vi "Create Tags.vi"(8 "error in (no error)":errorcluster, 9 "Module Tags Array Cluster":T1, 10 "folder node ID":T14, 11 "Refnum in":T17) -> (0 "error out":errorcluster, 3 "Tags Array":T16(array[cluster]))   [LabVIEW 2018]
uses:
  <vilib>/OPCUA/controls/OPC UA Server Refnum.ctl
  <vilib>/OPCUA/controls/NodeId.ctl
  <vilib>/OPCUA/controls/OPC UA Variable Node Refnum.ctl
  Module Tags Array Cluster.ctl
  Feed Module/Controls/Feed Module Tag Names Cluster.ctl
  TT Module/Controls/TT Module Tag Names.ctl
  PT Module/Controls/PT Module Tag Names.ctl
  Pump Module Folder/Pump Module Tag Names Cluster.ctl
  Bronkhorst M14 Flow Meter/Tag Cluster.ctl
  TCU Module/TCU Module Folder/TCU Module Tag Names Cluster.ctl
  D-O Module Folder/D-O Module Tag Names Cluster.ctl
  Pressure Regulator Control Module/Pressure Regulator/Controls/4-20mA Module Tag Names Cluster.ctl
  OPC Module Tag Names.ctl
  Sonicator Module Folder/Feed Module/Controls/Sonicator Module Tag Names.ctl
  Agitator Class/Agitator Module Tag Names.ctl
  Centrifuge Module Folder/Centrifuge Module Tag Names Cluster.ctl
  <vilib>/OPCUA/controls/Data Type.ctl
  <vilib>/regexp/Match Regular Expression.xnode
  <vilib>/OPCUA/NI OPC UA Server.lvlib
  Feed Module/Feed Module.lvlib
  Pump Module Folder/Pump Module.lvlib
  Flow Module Folder/Flow Module.lvlib
  TCU Module/TCU Module Folder/TCU Module.lvlib
  Pressure Regulator Control Module/Pressure Regulator/4-20mA Module.lvlib
  Sonicator Module Folder/Sonicator Module.lvlib
  Agitator Module Folder/Agitator Module.lvlib
  PT Module/PT Module.lvlib
  TT Module/TT Module.lvlib
  D-O Module Folder/D-O Module.lvlib
  Centrifuge Module Folder/Centrifuge Module.lvlib
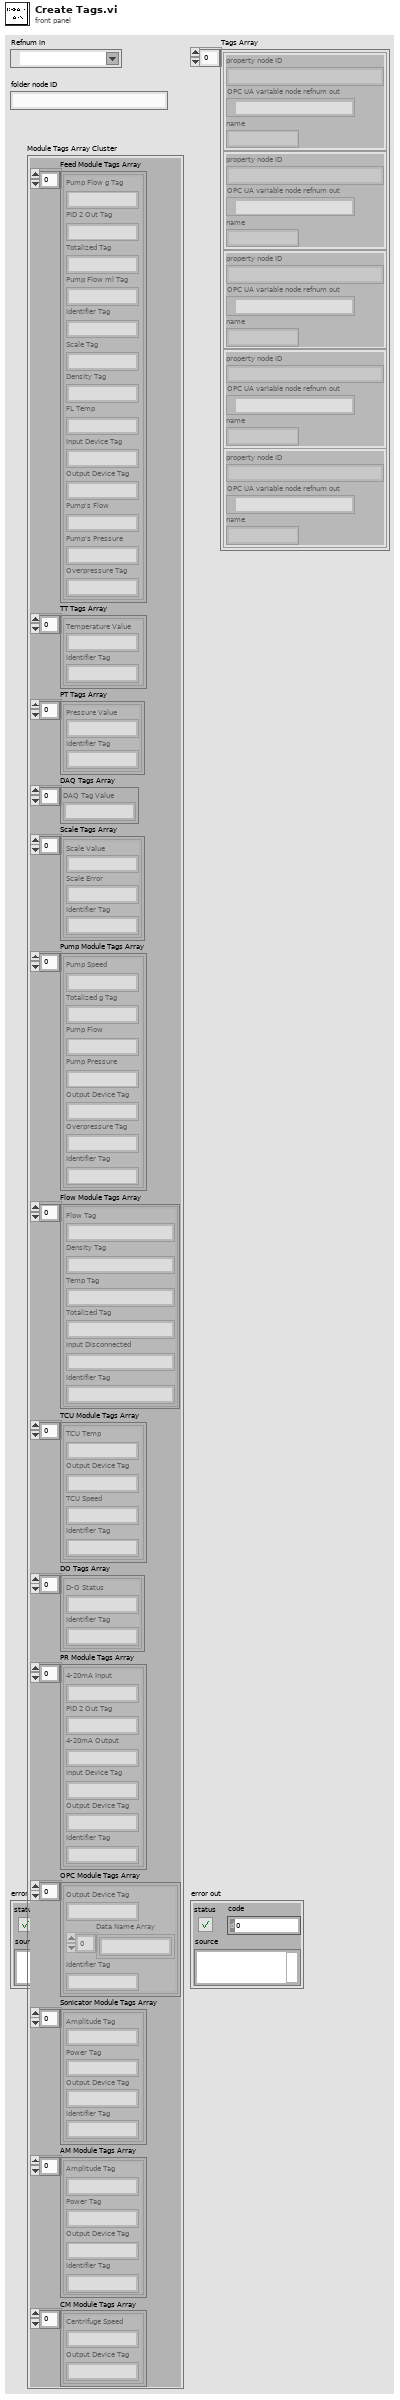
[diagram p1: front panel]
types:
  T1 = typedef "Module Tags Array Cluster.ctl" = cluster{"Feed Module Tags Array":T2[], "TT Tags Array":T3[], "PT Tags Array":T4[], "DAQ Tags Array":string[], "Scale Tags Array":cluster{"Scale Value":string, "Scale Error":string, "Identifier Tag":string}[], "Pump Module Tags Array":T5[], "Flow Module Tags Array":T6[], "TCU Module Tags Array":T7[], "DO Tags Array":T8[], "PR Module Tags Array":T9[], "OPC Module Tags Array":T10[], "Sonicator Module Tags Array":T11[], "AM Module Tags Array":T12[], "CM Module Tags Array":T13[]}
  T2 = typedef "Feed Module.lvlib/Feed Module Tag Names Cluster.ctl" = cluster{"Pump Flow g Tag":string, "PID 2 Out Tag":string, "Totalized Tag":string, "Pump Flow ml Tag":string, "Identifier Tag":string, "Scale Tag":string, "Density Tag":string, "FL Temp":string, "Input Device Tag":string, "Output Device Tag":string, "Pump's Flow":string, "Pump's Pressure":string, "Overpressure Tag":string}
  T3 = typedef "TT Module.lvlib/TT Module Tag Names.ctl" = cluster{"Temperature Value":string, "Identifier Tag":string}
  T4 = typedef "PT Module.lvlib/PT Module Tag Names.ctl" = cluster{"Pressure Value":string, "Identifier Tag":string}
  T5 = typedef "Pump Module.lvlib/Pump Module Tag Names Cluster.ctl" = cluster{"Pump Speed":string, "Totalized g Tag":string, "Pump Flow":string, "Pump Pressure":string, "Output Device Tag":string, "Overpressure Tag":string, "Identifier Tag":string}
  T6 = typedef "Flow Module.lvlib/Tag Cluster.ctl" = cluster{"Flow Tag":string, "Density Tag":string, "Temp Tag":string, "Totalized Tag":string, "Input Disconnected":string, "Identifier Tag":string}
  T7 = typedef "TCU Module.lvlib/TCU Module Tag Names Cluster.ctl" = cluster{"TCU Temp":string, "Output Device Tag":string, "TCU Speed":string, "Identifier Tag":string}
  T8 = typedef "D-O Module.lvlib/D-O Module Tag Names Cluster.ctl" = cluster{"D-O Status":string, "Identifier Tag":string}
  T9 = typedef "4-20mA Module.lvlib/4-20mA Module Tag Names Cluster.ctl" = cluster{"4-20mA Input":string, "PID 2 Out Tag":string, "4-20mA Output":string, "Input Device Tag":string, "Output Device Tag":string, "Identifier Tag":string}
  T10 = typedef "OPC Module Tag Names.ctl" = cluster{"Output Device Tag":string, "Data Name Array":string[], "Identifier Tag":string}
  T11 = typedef "Sonicator Module.lvlib/Sonicator Module Tag Names.ctl" = cluster{"Amplitude Tag":string, "Power Tag":string, "Output Device Tag":string, "Identifier Tag":string}
  T12 = typedef "Agitator Module.lvlib/Agitator Module Tag Names.ctl" = cluster{"Amplitude Tag":string, "Power Tag":string, "Output Device Tag":string, "Identifier Tag":string}
  T13 = typedef "Centrifuge Module.lvlib/Centrifuge Module Tag Names Cluster.ctl" = cluster{"Centrifuge Speed":string, "Output Device Tag":string}
  T14 = typedef "NodeId.ctl" = string
  T15 = typedef "OPC UA Variable Node Refnum.ctl" = refnum<k21>
  T16 = cluster{"property node ID":T14, "OPC UA variable node refnum out":T15, "name":string}[]
  T17 = typedef "OPC UA Server Refnum.ctl" = refnum<k21>
  T18 = cluster{"Scale Value":string, "Scale Error":string, "Identifier Tag":string}[]
  T19 = cluster{"property node ID":T14, "OPC UA variable node refnum out":T15, "name":string}
  T20 = typedef "Data Type.ctl" = u16
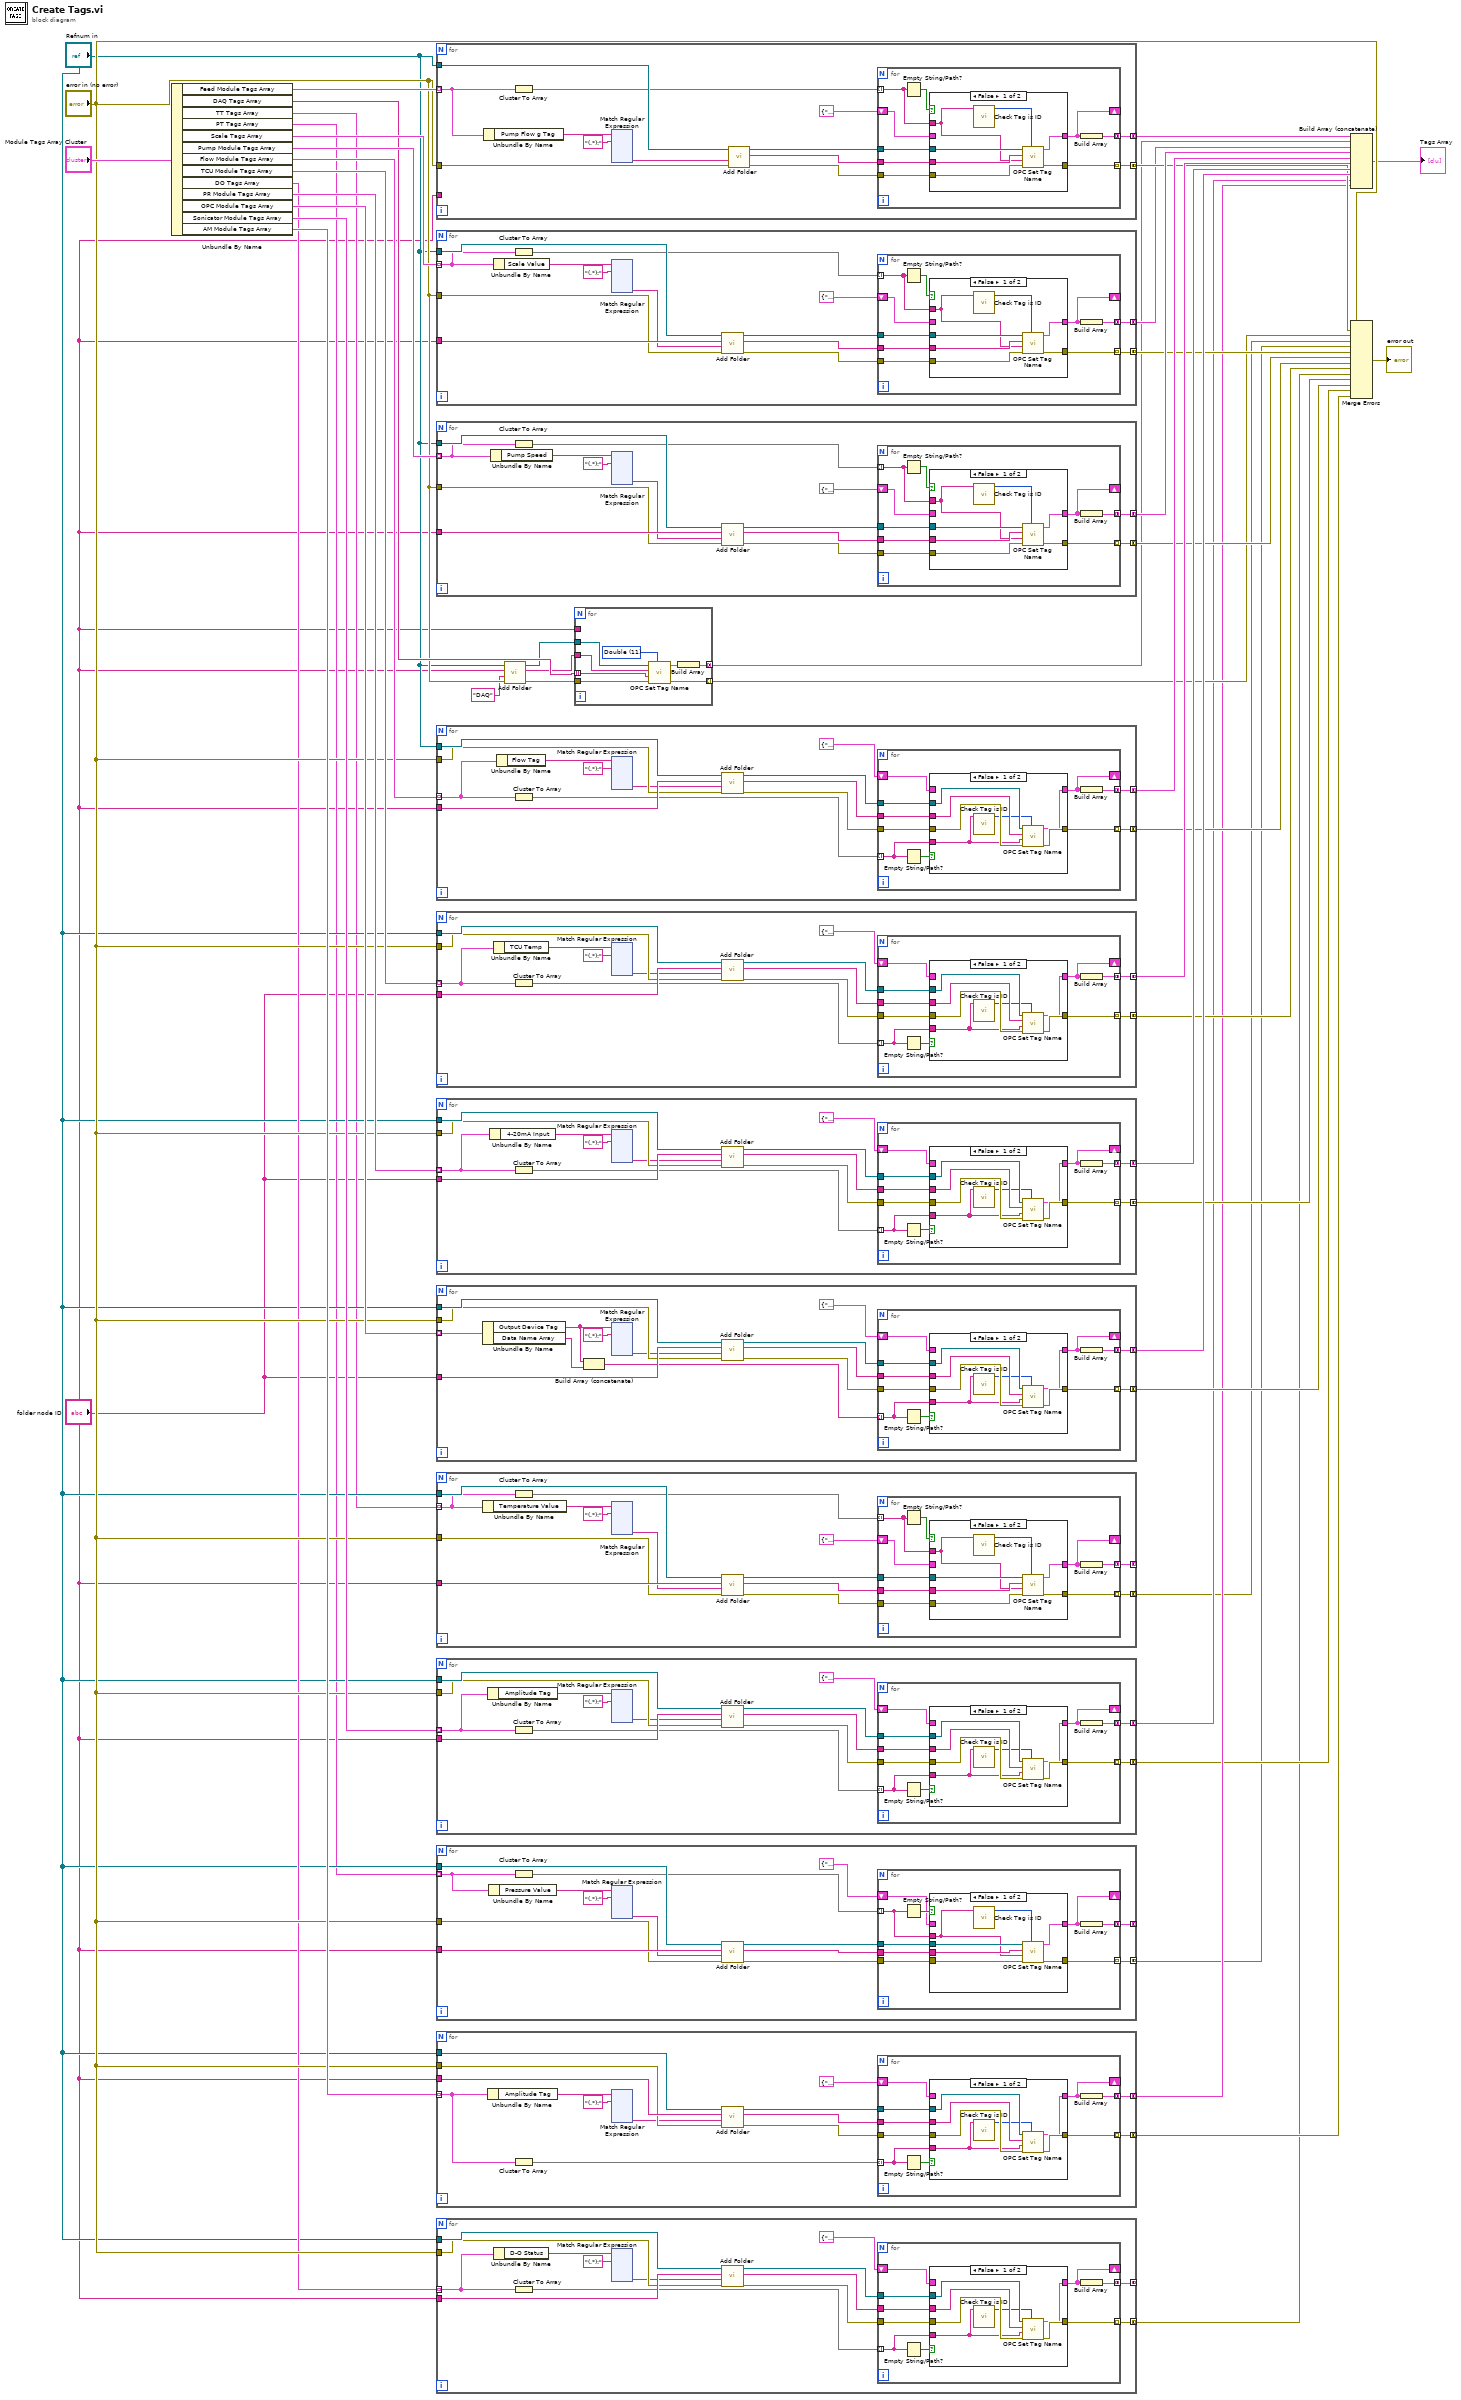
[diagram p0: block diagram]
diagram:
  n1 = Unbundle By Name("Module Tags Array Cluster") -> ("Feed Module Tags Array"=w22:T2[], "DAQ Tags Array"=w23:string[], "TT Tags Array"=w10:T3[], "PT Tags Array"=w11:T4[], "Scale Tags Array"=w25:T18, "Pump Module Tags Array"=w32:T5[], "Flow Module Tags Array"=w35:T6[], "TCU Module Tags Array"=w38:T7[], "DO Tags Array"=w13:T8[], "PR Module Tags Array"=w43:T9[], "OPC Module Tags Array"=w44:T10[], "Sonicator Module Tags Array"=w21:T11[], "AM Module Tags Array"=w20:T12[])
  n2 = for {
    tunnel: "error in (no error)" -> [w59]
    tunnel: "folder node ID" -> [_]
    tunnel: "Refnum in" -> [w58]
    tunnel: [w49] -> w30 mode=concatenating
    tunnel: w22 -> [w54] mode=indexing
    tunnel: [w47] -> w26 mode=concatenating
    n3 = Unbundle By Name(w54) -> ("Pump Flow g Tag"=w56:string)
    n4 = Cluster To Array(cluster=w54) -> (array=w53:string[])
    n5 = xnode "Match Regular Expression"("input string"=w56, "regular expression"="(.*):") -> ("submatch 1"=w55:string)  [unwired: 4 in, 5 out]
    n6 = call <vilib>:"Add Folder.vi"("error in (no error)"=w59, "folder name"=w55, "OPC UA server refnum in"=w58) -> ("error out"=w50:errorcluster, "folder node ID"=w52:T14, "OPC UA server refnum out"=w51:T17)  [unwired: 5 in]
    n7 = for {
      tunnel: w53 -> [w63] mode=indexing
      tunnel: w52 -> [w68]
      tunnel: w50 -> [w67]
      tunnel: w51 -> [w66]
      tunnel: [w65] -> w49 mode=indexing
      shift-right: [w61] -> _
      shift-left: T19 {"property node ID"="", "OPC UA variable node refnum out"="", "name"=""} ("OPC Property cluster") -> [w62]
      tunnel: [w60] -> w47 mode=concatenating
      n8 = Empty String/Path?(string/path=w63) -> (empty?=w64:bool)
      n9 = case shown="False" w64 {
        tunnel: w68 -> [w75 _]
        tunnel: w63 -> [w70 _]
        tunnel: w67 -> [w74 w77]
        tunnel: w66 -> [w73 _]
        tunnel: [w72 w77] -> w65
        tunnel: [w71 w76] -> w61
        tunnel: w62 -> [_ w76]
        frame False {
          n10 = call "Check Tag is ID.vi"("input string"=w70) -> ("data type"=w69:T20)  [unwired: 10 in]
          n11 = call "OPC Set Tag Name.vi"("data type"=w69, "error in (no error)"=w74, "name"=w70, "item node ID"=w75, "Refnum in"=w73) -> ("error out"=w72:errorcluster, "OPC Property cluster"=w71:T19)  [unwired: 5 in]
        }
        frame True {
        }
      }
      n12 = Build Array(w61) -> (w60:T16)
    }
  }
  n13 = for {
    tunnel: [w197] -> w31 mode=concatenating
    tunnel: w25 -> [w195] mode=indexing
    tunnel: "Refnum in" -> [w207]
    tunnel: "folder node ID" -> [w206]
    tunnel: "error in (no error)" -> [w205]
    tunnel: [w196] -> w28 mode=concatenating
    n14 = Unbundle By Name(w195) -> ("Scale Value"=w194:string)
    n15 = Cluster To Array(cluster=w195) -> (array=w202:string[])
    n16 = xnode "Match Regular Expression"("input string"=w194, "regular expression"="(.*):") -> ("submatch 1"=w203:string)  [unwired: 4 in, 5 out]
    n17 = call <vilib>:"Add Folder.vi"("error in (no error)"=w205, "folder name"=w203, "parent folder node ID"=w206, "OPC UA server refnum in"=w207) -> ("error out"=w200:errorcluster, "folder node ID"=w198:T14, "OPC UA server refnum out"=w199:T17)  [unwired: 4 in]
    n18 = for {
      tunnel: w202 -> [w211] mode=indexing
      tunnel: w198 -> [w216]
      tunnel: w200 -> [w215]
      tunnel: w199 -> [w214]
      tunnel: [w213] -> w197 mode=indexing
      shift-right: [w209] -> _
      shift-left: T19 {"property node ID"="", "OPC UA variable node refnum out"="", "name"=""} ("OPC Property cluster") -> [w210]
      tunnel: [w208] -> w196 mode=concatenating
      n19 = Empty String/Path?(string/path=w211) -> (empty?=w212:bool)
      n20 = case shown="False" w212 {
        tunnel: w216 -> [w223 _]
        tunnel: w211 -> [w218 _]
        tunnel: w215 -> [w222 w225]
        tunnel: w214 -> [w221 _]
        tunnel: [w220 w225] -> w213
        tunnel: [w219 w224] -> w209
        tunnel: w210 -> [_ w224]
        frame False {
          n21 = call "Check Tag is ID.vi"("input string"=w218) -> ("data type"=w217:T20)  [unwired: 10 in]
          n22 = call "OPC Set Tag Name.vi"("data type"=w217, "error in (no error)"=w222, "name"=w218, "item node ID"=w223, "Refnum in"=w221) -> ("error out"=w220:errorcluster, "OPC Property cluster"=w219:T19)  [unwired: 5 in]
        }
        frame True {
        }
      }
      n23 = Build Array(w209) -> (w208:T16)
    }
  }
  n24 = for {
    tunnel: [w345] -> w33 mode=concatenating
    tunnel: w32 -> [w343] mode=indexing
    tunnel: "Refnum in" -> [w355]
    tunnel: "folder node ID" -> [w354]
    tunnel: "error in (no error)" -> [w353]
    tunnel: [w344] -> w34 mode=concatenating
    n25 = Unbundle By Name(w343) -> ("Pump Speed"=w342:string)
    n26 = Cluster To Array(cluster=w343) -> (array=w350:string[])
    n27 = xnode "Match Regular Expression"("input string"=w342, "regular expression"="(.*):") -> ("submatch 1"=w351:string)  [unwired: 4 in, 5 out]
    n28 = call <vilib>:"Add Folder.vi"("error in (no error)"=w353, "folder name"=w351, "parent folder node ID"=w354, "OPC UA server refnum in"=w355) -> ("error out"=w348:errorcluster, "folder node ID"=w346:T14, "OPC UA server refnum out"=w347:T17)  [unwired: 4 in]
    n29 = for {
      tunnel: w350 -> [w359] mode=indexing
      tunnel: w346 -> [w364]
      tunnel: w348 -> [w363]
      tunnel: w347 -> [w362]
      tunnel: [w361] -> w345 mode=indexing
      shift-right: [w357] -> _
      shift-left: T19 {"property node ID"="", "OPC UA variable node refnum out"="", "name"=""} ("OPC Property cluster") -> [w358]
      tunnel: [w356] -> w344 mode=concatenating
      n30 = Empty String/Path?(string/path=w359) -> (empty?=w360:bool)
      n31 = case shown="False" w360 {
        tunnel: w364 -> [w371 _]
        tunnel: w359 -> [w366 _]
        tunnel: w363 -> [w370 w373]
        tunnel: w362 -> [w369 _]
        tunnel: [w368 w373] -> w361
        tunnel: [w367 w372] -> w357
        tunnel: w358 -> [_ w372]
        frame False {
          n32 = call "Check Tag is ID.vi"("input string"=w366) -> ("data type"=w365:T20)  [unwired: 10 in]
          n33 = call "OPC Set Tag Name.vi"("data type"=w365, "error in (no error)"=w370, "name"=w366, "item node ID"=w371, "Refnum in"=w369) -> ("error out"=w368:errorcluster, "OPC Property cluster"=w367:T19)  [unwired: 5 in]
        }
        frame True {
        }
      }
      n34 = Build Array(w357) -> (w356:T16)
    }
  }
  n35 = for {
    tunnel: [w493] -> w37 mode=concatenating
    tunnel: w35 -> [w491] mode=indexing
    tunnel: "Refnum in" -> [w503]
    tunnel: "folder node ID" -> [w502]
    tunnel: "error in (no error)" -> [w501]
    tunnel: [w492] -> w36 mode=concatenating
    n36 = Unbundle By Name(w491) -> ("Flow Tag"=w490:string)
    n37 = Cluster To Array(cluster=w491) -> (array=w498:string[])
    n38 = xnode "Match Regular Expression"("input string"=w490, "regular expression"="(.*):") -> ("submatch 1"=w499:string)  [unwired: 4 in, 5 out]
    n39 = call <vilib>:"Add Folder.vi"("error in (no error)"=w501, "folder name"=w499, "parent folder node ID"=w502, "OPC UA server refnum in"=w503) -> ("error out"=w496:errorcluster, "folder node ID"=w494:T14, "OPC UA server refnum out"=w495:T17)  [unwired: 4 in]
    n40 = for {
      tunnel: w498 -> [w507] mode=indexing
      tunnel: w494 -> [w512]
      tunnel: w496 -> [w511]
      tunnel: w495 -> [w510]
      tunnel: [w509] -> w493 mode=indexing
      shift-right: [w505] -> _
      shift-left: T19 {"property node ID"="", "OPC UA variable node refnum out"="", "name"=""} ("OPC Property cluster") -> [w506]
      tunnel: [w504] -> w492 mode=concatenating
      n41 = Empty String/Path?(string/path=w507) -> (empty?=w508:bool)
      n42 = case shown="False" w508 {
        tunnel: w512 -> [w519 _]
        tunnel: w507 -> [w514 _]
        tunnel: w511 -> [w518 w521]
        tunnel: w510 -> [w517 _]
        tunnel: [w516 w521] -> w509
        tunnel: [w515 w520] -> w505
        tunnel: w506 -> [_ w520]
        frame False {
          n43 = call "Check Tag is ID.vi"("input string"=w514) -> ("data type"=w513:T20)  [unwired: 10 in]
          n44 = call "OPC Set Tag Name.vi"("data type"=w513, "error in (no error)"=w518, "name"=w514, "item node ID"=w519, "Refnum in"=w517) -> ("error out"=w516:errorcluster, "OPC Property cluster"=w515:T19)  [unwired: 5 in]
        }
        frame True {
        }
      }
      n45 = Build Array(w505) -> (w504:T16)
    }
  }
  n46 = for {
    tunnel: [w641] -> w39 mode=concatenating
    tunnel: w38 -> [w639] mode=indexing
    tunnel: "Refnum in" -> [w651]
    tunnel: "folder node ID" -> [w650]
    tunnel: "error in (no error)" -> [w649]
    tunnel: [w640] -> w40 mode=concatenating
    n47 = Unbundle By Name(w639) -> ("TCU Temp"=w638:string)
    n48 = Cluster To Array(cluster=w639) -> (array=w646:string[])
    n49 = xnode "Match Regular Expression"("input string"=w638, "regular expression"="(.*):") -> ("submatch 1"=w647:string)  [unwired: 4 in, 5 out]
    n50 = call <vilib>:"Add Folder.vi"("error in (no error)"=w649, "folder name"=w647, "parent folder node ID"=w650, "OPC UA server refnum in"=w651) -> ("error out"=w644:errorcluster, "folder node ID"=w642:T14, "OPC UA server refnum out"=w643:T17)  [unwired: 4 in]
    n51 = for {
      tunnel: w646 -> [w655] mode=indexing
      tunnel: w642 -> [w660]
      tunnel: w644 -> [w659]
      tunnel: w643 -> [w658]
      tunnel: [w657] -> w641 mode=indexing
      shift-right: [w653] -> _
      shift-left: T19 {"property node ID"="", "OPC UA variable node refnum out"="", "name"=""} ("OPC Property cluster") -> [w654]
      tunnel: [w652] -> w640 mode=concatenating
      n52 = Empty String/Path?(string/path=w655) -> (empty?=w656:bool)
      n53 = case shown="False" w656 {
        tunnel: w660 -> [w667 _]
        tunnel: w655 -> [w662 _]
        tunnel: w659 -> [w666 w669]
        tunnel: w658 -> [w665 _]
        tunnel: [w664 w669] -> w657
        tunnel: [w663 w668] -> w653
        tunnel: w654 -> [_ w668]
        frame False {
          n54 = call "Check Tag is ID.vi"("input string"=w662) -> ("data type"=w661:T20)  [unwired: 10 in]
          n55 = call "OPC Set Tag Name.vi"("data type"=w661, "error in (no error)"=w666, "name"=w662, "item node ID"=w667, "Refnum in"=w665) -> ("error out"=w664:errorcluster, "OPC Property cluster"=w663:T19)  [unwired: 5 in]
        }
        frame True {
        }
      }
      n56 = Build Array(w653) -> (w652:T16)
    }
  }
  n57 = for {
    tunnel: [w789] -> w41 mode=concatenating
    tunnel: w43 -> [w787] mode=indexing
    tunnel: "Refnum in" -> [w799]
    tunnel: "folder node ID" -> [w798]
    tunnel: "error in (no error)" -> [w797]
    tunnel: [w788] -> w42 mode=concatenating
    n58 = Unbundle By Name(w787) -> ("4-20mA Input"=w786:string)
    n59 = Cluster To Array(cluster=w787) -> (array=w794:string[])
    n60 = xnode "Match Regular Expression"("input string"=w786, "regular expression"="(.*):") -> ("submatch 1"=w795:string)  [unwired: 4 in, 5 out]
    n61 = call <vilib>:"Add Folder.vi"("error in (no error)"=w797, "folder name"=w795, "parent folder node ID"=w798, "OPC UA server refnum in"=w799) -> ("error out"=w792:errorcluster, "folder node ID"=w790:T14, "OPC UA server refnum out"=w791:T17)  [unwired: 4 in]
    n62 = for {
      tunnel: w794 -> [w803] mode=indexing
      tunnel: w790 -> [w808]
      tunnel: w792 -> [w807]
      tunnel: w791 -> [w806]
      tunnel: [w805] -> w789 mode=indexing
      shift-right: [w801] -> _
      shift-left: T19 {"property node ID"="", "OPC UA variable node refnum out"="", "name"=""} ("OPC Property cluster") -> [w802]
      tunnel: [w800] -> w788 mode=concatenating
      n63 = Empty String/Path?(string/path=w803) -> (empty?=w804:bool)
      n64 = case shown="False" w804 {
        tunnel: w808 -> [w815 _]
        tunnel: w803 -> [w810 _]
        tunnel: w807 -> [w814 w817]
        tunnel: w806 -> [w813 _]
        tunnel: [w812 w817] -> w805
        tunnel: [w811 w816] -> w801
        tunnel: w802 -> [_ w816]
        frame False {
          n65 = call "Check Tag is ID.vi"("input string"=w810) -> ("data type"=w809:T20)  [unwired: 10 in]
          n66 = call "OPC Set Tag Name.vi"("data type"=w809, "error in (no error)"=w814, "name"=w810, "item node ID"=w815, "Refnum in"=w813) -> ("error out"=w812:errorcluster, "OPC Property cluster"=w811:T19)  [unwired: 5 in]
        }
        frame True {
        }
      }
      n67 = Build Array(w801) -> (w800:T16)
    }
  }
  n68 = for {
    tunnel: [w939] -> w45 mode=concatenating
    tunnel: w44 -> [w937] mode=indexing
    tunnel: "Refnum in" -> [w948]
    tunnel: "folder node ID" -> [w947]
    tunnel: "error in (no error)" -> [w946]
    tunnel: [w938] -> w46 mode=concatenating
    n69 = Unbundle By Name(w937) -> ("Output Device Tag"=w936:string, "Data Name Array"=w935:string[])
    n70 = Build Array (concatenate)(w936, w935) -> (w934:string[])
    n71 = xnode "Match Regular Expression"("input string"=w936, "regular expression"="(.*):") -> ("submatch 1"=w944:string)  [unwired: 4 in, 5 out]
    n72 = call <vilib>:"Add Folder.vi"("error in (no error)"=w946, "folder name"=w944, "parent folder node ID"=w947, "OPC UA server refnum in"=w948) -> ("error out"=w942:errorcluster, "folder node ID"=w940:T14, "OPC UA server refnum out"=w941:T17)  [unwired: 4 in]
    n73 = for {
      tunnel: w934 -> [w952] mode=indexing
      tunnel: w940 -> [w957]
      tunnel: w942 -> [w956]
      tunnel: w941 -> [w955]
      tunnel: [w954] -> w939 mode=indexing
      shift-right: [w950] -> _
      shift-left: T19 {"property node ID"="", "OPC UA variable node refnum out"="", "name"=""} ("OPC Property cluster") -> [w951]
      tunnel: [w949] -> w938 mode=concatenating
      n74 = Empty String/Path?(string/path=w952) -> (empty?=w953:bool)
      n75 = case shown="False" w953 {
        tunnel: w957 -> [w964 _]
        tunnel: w952 -> [w959 _]
        tunnel: w956 -> [w963 w966]
        tunnel: w955 -> [w962 _]
        tunnel: [w961 w966] -> w954
        tunnel: [w960 w965] -> w950
        tunnel: w951 -> [_ w965]
        frame False {
          n76 = call "Check Tag is ID.vi"("input string"=w959) -> ("data type"=w958:T20)  [unwired: 10 in]
          n77 = call "OPC Set Tag Name.vi"("data type"=w958, "error in (no error)"=w963, "name"=w959, "item node ID"=w964, "Refnum in"=w962) -> ("error out"=w961:errorcluster, "OPC Property cluster"=w960:T19)  [unwired: 5 in]
        }
        frame True {
        }
      }
      n78 = Build Array(w950) -> (w949:T16)
    }
  }
  n79 = for {
    tunnel: [w1086] -> w9 mode=concatenating
    tunnel: w10 -> [w1084] mode=indexing
    tunnel: "Refnum in" -> [w1096]
    tunnel: "folder node ID" -> [w1095]
    tunnel: "error in (no error)" -> [w1094]
    tunnel: [w1085] -> _ mode=concatenating
    n80 = Unbundle By Name(w1084) -> ("Temperature Value"=w1083:string)
    n81 = Cluster To Array(cluster=w1084) -> (array=w1091:string[])
    n82 = xnode "Match Regular Expression"("input string"=w1083, "regular expression"="(.*):") -> ("submatch 1"=w1092:string)  [unwired: 4 in, 5 out]
    n83 = call <vilib>:"Add Folder.vi"("error in (no error)"=w1094, "folder name"=w1092, "parent folder node ID"=w1095, "OPC UA server refnum in"=w1096) -> ("error out"=w1089:errorcluster, "folder node ID"=w1087:T14, "OPC UA server refnum out"=w1088:T17)  [unwired: 4 in]
    n84 = for {
      tunnel: w1091 -> [w1100] mode=indexing
      tunnel: w1087 -> [w1105]
      tunnel: w1089 -> [w1104]
      tunnel: w1088 -> [w1103]
      tunnel: [w1102] -> w1086 mode=indexing
      shift-right: [w1098] -> _
      shift-left: T19 {"property node ID"="", "OPC UA variable node refnum out"="", "name"=""} ("OPC Property cluster") -> [w1099]
      tunnel: [w1097] -> w1085 mode=concatenating
      n85 = Empty String/Path?(string/path=w1100) -> (empty?=w1101:bool)
      n86 = case shown="False" w1101 {
        tunnel: w1105 -> [w1112 _]
        tunnel: w1100 -> [w1107 _]
        tunnel: w1104 -> [w1111 w1114]
        tunnel: w1103 -> [w1110 _]
        tunnel: [w1109 w1114] -> w1102
        tunnel: [w1108 w1113] -> w1098
        tunnel: w1099 -> [_ w1113]
        frame False {
          n87 = call "Check Tag is ID.vi"("input string"=w1107) -> ("data type"=w1106:T20)  [unwired: 10 in]
          n88 = call "OPC Set Tag Name.vi"("data type"=w1106, "error in (no error)"=w1111, "name"=w1107, "item node ID"=w1112, "Refnum in"=w1110) -> ("error out"=w1109:errorcluster, "OPC Property cluster"=w1108:T19)  [unwired: 5 in]
        }
        frame True {
        }
      }
      n89 = Build Array(w1098) -> (w1097:T16)
    }
  }
  n90 = for {
    tunnel: [w1234] -> w17 mode=concatenating
    tunnel: w21 -> [w1232] mode=indexing
    tunnel: "Refnum in" -> [w1244]
    tunnel: "folder node ID" -> [w1243]
    tunnel: "error in (no error)" -> [w1242]
    tunnel: [w1233] -> w19 mode=concatenating
    n91 = Unbundle By Name(w1232) -> ("Amplitude Tag"=w1231:string)
    n92 = Cluster To Array(cluster=w1232) -> (array=w1239:string[])
    n93 = xnode "Match Regular Expression"("input string"=w1231, "regular expression"="(.*):") -> ("submatch 1"=w1240:string)  [unwired: 4 in, 5 out]
    n94 = call <vilib>:"Add Folder.vi"("error in (no error)"=w1242, "folder name"=w1240, "parent folder node ID"=w1243, "OPC UA server refnum in"=w1244) -> ("error out"=w1237:errorcluster, "folder node ID"=w1235:T14, "OPC UA server refnum out"=w1236:T17)  [unwired: 4 in]
    n95 = for {
      tunnel: w1239 -> [w1248] mode=indexing
      tunnel: w1235 -> [w1253]
      tunnel: w1237 -> [w1252]
      tunnel: w1236 -> [w1251]
      tunnel: [w1250] -> w1234 mode=indexing
      shift-right: [w1246] -> _
      shift-left: T19 {"property node ID"="", "OPC UA variable node refnum out"="", "name"=""} ("OPC Property cluster") -> [w1247]
      tunnel: [w1245] -> w1233 mode=concatenating
      n96 = Empty String/Path?(string/path=w1248) -> (empty?=w1249:bool)
      n97 = case shown="False" w1249 {
        tunnel: w1253 -> [w1260 _]
        tunnel: w1248 -> [w1255 _]
        tunnel: w1252 -> [w1259 w1262]
        tunnel: w1251 -> [w1258 _]
        tunnel: [w1257 w1262] -> w1250
        tunnel: [w1256 w1261] -> w1246
        tunnel: w1247 -> [_ w1261]
        frame False {
          n98 = call "Check Tag is ID.vi"("input string"=w1255) -> ("data type"=w1254:T20)  [unwired: 10 in]
          n99 = call "OPC Set Tag Name.vi"("data type"=w1254, "error in (no error)"=w1259, "name"=w1255, "item node ID"=w1260, "Refnum in"=w1258) -> ("error out"=w1257:errorcluster, "OPC Property cluster"=w1256:T19)  [unwired: 5 in]
        }
        frame True {
        }
      }
      n100 = Build Array(w1246) -> (w1245:T16)
    }
  }
  n101 = for {
    tunnel: [w1382] -> w8 mode=concatenating
    tunnel: w11 -> [w1380] mode=indexing
    tunnel: "Refnum in" -> [w1392]
    tunnel: "folder node ID" -> [w1391]
    tunnel: "error in (no error)" -> [w1390]
    tunnel: [w1381] -> _ mode=concatenating
    n102 = Unbundle By Name(w1380) -> ("Pressure Value"=w1379:string)
    n103 = Cluster To Array(cluster=w1380) -> (array=w1387:string[])
    n104 = xnode "Match Regular Expression"("input string"=w1379, "regular expression"="(.*):") -> ("submatch 1"=w1388:string)  [unwired: 4 in, 5 out]
    n105 = call <vilib>:"Add Folder.vi"("error in (no error)"=w1390, "folder name"=w1388, "parent folder node ID"=w1391, "OPC UA server refnum in"=w1392) -> ("error out"=w1385:errorcluster, "folder node ID"=w1383:T14, "OPC UA server refnum out"=w1384:T17)  [unwired: 4 in]
    n106 = for {
      tunnel: w1387 -> [w1396] mode=indexing
      tunnel: w1383 -> [w1401]
      tunnel: w1385 -> [w1400]
      tunnel: w1384 -> [w1399]
      tunnel: [w1398] -> w1382 mode=indexing
      shift-right: [w1394] -> _
      shift-left: T19 {"property node ID"="", "OPC UA variable node refnum out"="", "name"=""} ("OPC Property cluster") -> [w1395]
      tunnel: [w1393] -> w1381 mode=concatenating
      n107 = Empty String/Path?(string/path=w1396) -> (empty?=w1397:bool)
      n108 = case shown="False" w1397 {
        tunnel: w1401 -> [w1408 _]
        tunnel: w1396 -> [w1403 _]
        tunnel: w1400 -> [w1407 w1410]
        tunnel: w1399 -> [w1406 _]
        tunnel: [w1405 w1410] -> w1398
        tunnel: [w1404 w1409] -> w1394
        tunnel: w1395 -> [_ w1409]
        frame False {
          n109 = call "Check Tag is ID.vi"("input string"=w1403) -> ("data type"=w1402:T20)  [unwired: 10 in]
          n110 = call "OPC Set Tag Name.vi"("data type"=w1402, "error in (no error)"=w1407, "name"=w1403, "item node ID"=w1408, "Refnum in"=w1406) -> ("error out"=w1405:errorcluster, "OPC Property cluster"=w1404:T19)  [unwired: 5 in]
        }
        frame True {
        }
      }
      n111 = Build Array(w1394) -> (w1393:T16)
    }
  }
  n112 = for {
    tunnel: [w1530] -> w16 mode=concatenating
    tunnel: w20 -> [w1528] mode=indexing
    tunnel: "Refnum in" -> [w1540]
    tunnel: "folder node ID" -> [w1539]
    tunnel: "error in (no error)" -> [w1538]
    tunnel: [w1529] -> w18 mode=concatenating
    n113 = Unbundle By Name(w1528) -> ("Amplitude Tag"=w1527:string)
    n114 = Cluster To Array(cluster=w1528) -> (array=w1535:string[])
    n115 = xnode "Match Regular Expression"("input string"=w1527, "regular expression"="(.*):") -> ("submatch 1"=w1536:string)  [unwired: 4 in, 5 out]
    n116 = call <vilib>:"Add Folder.vi"("error in (no error)"=w1538, "folder name"=w1536, "parent folder node ID"=w1539, "OPC UA server refnum in"=w1540) -> ("error out"=w1533:errorcluster, "folder node ID"=w1531:T14, "OPC UA server refnum out"=w1532:T17)  [unwired: 4 in]
    n117 = for {
      tunnel: w1535 -> [w1544] mode=indexing
      tunnel: w1531 -> [w1549]
      tunnel: w1533 -> [w1548]
      tunnel: w1532 -> [w1547]
      tunnel: [w1546] -> w1530 mode=indexing
      shift-right: [w1542] -> _
      shift-left: T19 {"property node ID"="", "OPC UA variable node refnum out"="", "name"=""} ("OPC Property cluster") -> [w1543]
      tunnel: [w1541] -> w1529 mode=concatenating
      n118 = Empty String/Path?(string/path=w1544) -> (empty?=w1545:bool)
      n119 = case shown="False" w1545 {
        tunnel: w1549 -> [w1556 _]
        tunnel: w1544 -> [w1551 _]
        tunnel: w1548 -> [w1555 w1558]
        tunnel: w1547 -> [w1554 _]
        tunnel: [w1553 w1558] -> w1546
        tunnel: [w1552 w1557] -> w1542
        tunnel: w1543 -> [_ w1557]
        frame False {
          n120 = call "Check Tag is ID.vi"("input string"=w1551) -> ("data type"=w1550:T20)  [unwired: 10 in]
          n121 = call "OPC Set Tag Name.vi"("data type"=w1550, "error in (no error)"=w1555, "name"=w1551, "item node ID"=w1556, "Refnum in"=w1554) -> ("error out"=w1553:errorcluster, "OPC Property cluster"=w1552:T19)  [unwired: 5 in]
        }
        frame True {
        }
      }
      n122 = Build Array(w1542) -> (w1541:T16)
    }
  }
  n123 = for {
    tunnel: [w1678] -> w7 mode=concatenating
    tunnel: w13 -> [w1676] mode=indexing
    tunnel: "Refnum in" -> [w1688]
    tunnel: "folder node ID" -> [w1687]
    tunnel: "error in (no error)" -> [w1686]
    tunnel: [w1677] -> _ mode=concatenating
    n124 = Unbundle By Name(w1676) -> ("D-O Status"=w1675:string)
    n125 = Cluster To Array(cluster=w1676) -> (array=w1683:string[])
    n126 = xnode "Match Regular Expression"("input string"=w1675, "regular expression"="(.*):") -> ("submatch 1"=w1684:string)  [unwired: 4 in, 5 out]
    n127 = call <vilib>:"Add Folder.vi"("error in (no error)"=w1686, "folder name"=w1684, "parent folder node ID"=w1687, "OPC UA server refnum in"=w1688) -> ("error out"=w1681:errorcluster, "folder node ID"=w1679:T14, "OPC UA server refnum out"=w1680:T17)  [unwired: 4 in]
    n128 = for {
      tunnel: w1683 -> [w1692] mode=indexing
      tunnel: w1679 -> [w1697]
      tunnel: w1681 -> [w1696]
      tunnel: w1680 -> [w1695]
      tunnel: [w1694] -> w1678 mode=indexing
      shift-right: [w1690] -> _
      shift-left: T19 {"property node ID"="", "OPC UA variable node refnum out"="", "name"=""} ("OPC Property cluster") -> [w1691]
      tunnel: [w1689] -> w1677 mode=concatenating
      n129 = Empty String/Path?(string/path=w1692) -> (empty?=w1693:bool)
      n130 = case shown="False" w1693 {
        tunnel: w1697 -> [w1704 _]
        tunnel: w1692 -> [w1699 _]
        tunnel: w1696 -> [w1703 w1706]
        tunnel: w1695 -> [w1702 _]
        tunnel: [w1701 w1706] -> w1694
        tunnel: [w1700 w1705] -> w1690
        tunnel: w1691 -> [_ w1705]
        frame False {
          n131 = call "Check Tag is ID.vi"("input string"=w1699) -> ("data type"=w1698:T20)  [unwired: 10 in]
          n132 = call "OPC Set Tag Name.vi"("data type"=w1698, "error in (no error)"=w1703, "name"=w1699, "item node ID"=w1704, "Refnum in"=w1702) -> ("error out"=w1701:errorcluster, "OPC Property cluster"=w1700:T19)  [unwired: 5 in]
        }
        frame True {
        }
      }
      n133 = Build Array(w1690) -> (w1689:T16)
    }
  }
  n134 = call <vilib>:"Add Folder.vi"("error in (no error)"="error in (no error)", "folder name"="DAQ", "parent folder node ID"="folder node ID", "OPC UA server refnum in"="Refnum in") -> ("error out"=w4:errorcluster, "folder node ID"=w3:T14, "OPC UA server refnum out"=w2:T17)  [unwired: 4 in]
  n135 = for {
    tunnel: "folder node ID" -> [_]
    tunnel: [w1830] -> w29 mode=indexing
    tunnel: w23 -> [w1828] mode=indexing
    tunnel: [w1829] -> w27 mode=concatenating
    tunnel: w4 -> [w1825]
    tunnel: w3 -> [w1824]
    tunnel: w2 -> [w1823]
    w1826 = T20 11 items=["Boolean"=1, "SByte"=2, "Byte"=3, "Int16"=4, "UInt16"=5, "Int32"=6, "UInt32"=7, "Int64"=8, "UInt64"=9, "Float"=10, "Double"=11, "String"=12, "DateTime"=13, "ByteString"=15, "Array of Boolean"=101, "Array of SByte"=102, "Array of Byte"=103, "Array of Int16"=104, "Array of UInt16"=105, "Array of Int32"=106, "Array of UInt32"=107, "Array of Int64"=108, "Array of UInt64"=109, "Array of Float"=110, "Array of Double"=111, "Array of String"=112, "Array of DateTime"=113, "Array of ByteString"=115, "Matrix of Boolean"=201, "Matrix of SByte"=202, "Matrix of Byte"=203, "Matrix of Int16"=204, "Matrix of UInt16"=205, "Matrix of Int32"=206, "Matrix of UInt32"=207, "Matrix of Int64"=208, "Matrix of UInt64"=209, "Matrix of Float"=210, "Matrix of Double"=211, "Matrix of String "=212, "Matrix of DateTime"=213, "Matrix of ByteString"=215] ("data type")
    n136 = call "OPC Set Tag Name.vi"("data type"=w1826, "error in (no error)"=w1825, "name"=w1828, "item node ID"=w1824, "Refnum in"=w1823) -> ("error out"=w1830:errorcluster, "OPC Property cluster"=w1827:T19)  [unwired: 5 in]
    n137 = Build Array(w1827) -> (w1829:T16)
  }
  n138 = Build Array (concatenate)(w26, w27, w28, w34, w36, w40, w42, w46, w19, w18) -> (→"Tags Array":T16)
  n139 = Merge Errors("error in (no error)", w30, w29, w9, w8, w31, w33, w37, w39, w7, w41, w45, w17, w16) -> (→"error out":errorcluster)
